vi "Y DISPLACEMENT.vi"(1 "Desce ou sobe?":bool, 2 "Distância Ac (um)":dbl=50.0, 3 "Distância Guias (um)":dbl=50.0) -> (0 "Delta Y":dbl)   [LabVIEW 2014]
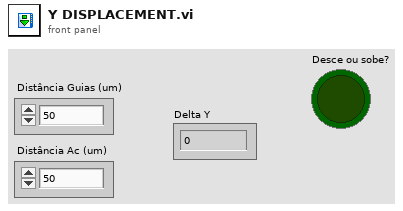
[diagram p1: front panel]
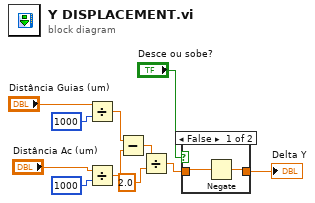
[diagram p0: block diagram]
diagram:
  n1 = Divide(x="Distância Guias (um)", y=1000) -> (x/y=w7:dbl)
  n2 = Divide(x="Distância Ac (um)", y=1000) -> (x/y=w6:dbl)
  n3 = Subtract(x=w7, y=w6) -> (x-y=w5:dbl)
  n4 = Divide(x=w5, y=2.0) -> (x/y=w2:dbl)
  n5 = case shown="False" "Desce ou sobe?" {
    tunnel: [w13 w14] -> w1
    tunnel: w2 -> [w12 w14]
    frame False {
      n6 = Negate(x=w12) -> (-x=w13:dbl)
    }
    frame True {
    }
  }
  "Delta Y" <- w1
